vi "创建数组.vi"() -> ()   [LabVIEW 2012]
panel:
  out "连接数组":i32[](array[numeric])
  out "合并数组":i32[][](array[numeric])
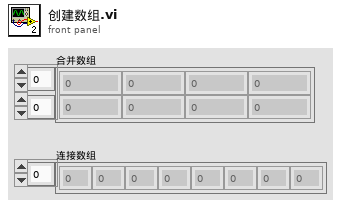
[diagram p1: front panel]
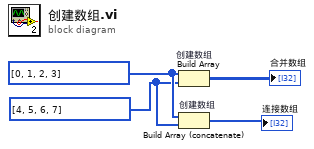
[diagram p0: block diagram]
diagram:
  w2 = i32[] [4, 5, 6, 7]
  w3 = i32[] [0, 1, 2, 3]
  n1 = Build Array "创建数组"(w3, w2) -> (→"合并数组":i32[][])
  n2 = Build Array (concatenate) "创建数组"(w3, w2) -> (→"连接数组":i32[])
